vi "edit1.vi"() -> ()   [LabVIEW 2017]
uses:
  <vilib>/userdefined/High Color/IMAQdx.ctl
  <vilib>/myRIO/Instrument Drivers/Onboard IO/DIO/typedefs/DIO Reference.ctl
  <vilib>/myRIO/Common/Instrument Driver Framework/Utilities/typedefs/myRIO Generic Hardware Reference.ctl
  <vilib>/myRIO/Common/Instrument Driver Framework/Utilities/typedefs/Hardware Version Enum.ctl
  <vilib>/myRIO/Common/Instrument Driver Framework/Utilities/typedefs/myRIO v1.0 Reference.ctl
  <vilib>/myRIO/Common/Instrument Driver Framework/Utilities/typedefs/Generic FPGA Reference.ctl
  <vilib>/myRIO/Common/Instrument Driver Framework/myRIO v1.0/DIO/typedefs/DIO Channels List.ctl
  <vilib>/myRIO/Common/Instrument Driver Framework/myRIO v1.0/DIO/typedefs/DIO Channels Enum.ctl
  <vilib>/userdefined/High Color/nirio_resource_hc.ctl
  <vilib>/Platform/TimedLoop/XDataNode/timing_clust.ctl
  <vilib>/Platform/TimedLoop/XDataNode/nitl_modes.ctl
  <vilib>/Platform/TimedLoop/XDataNode/wakeup.ctl
  <vilib>/myRIO/Common/Instrument Driver Framework/Utilities/vis/Is FPGA Ref Available.vi
  <vilib>/myRIO/Common/Instrument Driver Framework/myRIO v1.0/DIO/vis/myRIO v1.1 Open DIO.vi
  <vilib>/myRIO/Instrument Drivers/Onboard IO/DIO/vis/Read.vi
  <vilib>/myRIO/Common/Instrument Driver Framework/Utilities/vis/Validate Channels.vi
  <vilib>/myRIO/Common/Instrument Driver Framework/myRIO v1.0/DIO/vis/myRIO v1.0 Reserve DIO.vi
  <vilib>/myRIO/Common/Instrument Driver Framework/myRIO v1.0/UART/vis/myRIO v1.0 Close UART.vi
  <vilib>/myRIO/Common/Instrument Driver Framework/myRIO v1.0/Resource Manager/vis/myRIO v1.0 Reserve Channel List.vi
  <vilib>/myRIO/Common/Instrument Driver Framework/myRIO v1.0/DIO/vis/myRIO v1.0 Build MUX Configuration DIO.vi
  <vilib>/myRIO/Common/Instrument Driver Framework/myRIO v1.0/Resource Manager/vis/myRIO v1.0 Reserve Channel.vi
  <vilib>/myRIO/Common/Instrument Driver Framework/myRIO v1.0/Resource Manager/vis/myRIO v1.0 Unreserve Channel.vi
  <vilib>/myRIO/Common/Instrument Driver Framework/myRIO v1.0/Resource Manager/vis/myRIO v1.0 Create Configuration List.vi
  <vilib>/myRIO/Common/Instrument Driver Framework/myRIO v1.0/Resource Manager/vis/myRIO v1.0 Build Mutex Name.vi
  Global 1.vi
  Outputs.vi
  Inputs.vi
  <vilib>/Utility/VariantDataType/GetNumericInfo.vi
  <vilib>/Utility/error.llb/Error Cluster From Error Code.vi
  <vilib>/myRIO/Common/Instrument Driver Framework/myRIO v1.0/myRIO v1.1 Open.vi
  <vilib>/myRIO/Common/Instrument Driver Framework/Utilities/vis/IO Manager.vi
  <vilib>/myRIO/Common/Instrument Driver Framework/Utilities/vis/Configuration Manager.vi
  <vilib>/myRIO/Common/Instrument Driver Framework/myRIO v1.0/Resource Manager/vis/myRIO v1.0 Configure IO.vi
  <vilib>/myRIO/Common/Instrument Driver Framework/myRIO v1.0/myRIO v1.0 Close.vi
  <vilib>/myRIO/Common/Instrument Driver Framework/myRIO v1.0/DIO/vis/myRIO v1.0 Read DIO.vi
  <vilib>/myRIO/Common/Instrument Driver Framework/Utilities/vis/FPGA Ref Manager.vi
  <vilib>/myRIO/Common/Instrument Driver Framework/myRIO v1.0/myRIO v1.0 Reset FPGA.vi
  <vilib>/myRIO/Common/Instrument Driver Framework/myRIO v1.0/IRQ/vis/myRIO v1.0 IRQ Info FGV.vi
  <vilib>/myRIO/Common/Instrument Driver Framework/myRIO v1.0/IRQ/vis/myRIO v1.0 Timer IRQ Info FGV.vi
  <vilib>/myRIO/Common/Instrument Driver Framework/myRIO v1.0/IRQ/vis/myRIO v1.0 ISR Agent.vi
  <vilib>/myRIO/Express VI/Onboard IO/DI/DI Express VI.xnode
  <vilib>/myRIO/Instrument Drivers/Onboard IO/DIO/vis/myRIO DIO Open.xnode
  <vilib>/platform/TimedLoop/XDataNode/XDataNode.xnode
  <vilib>/vision/driver/NI_Vision_Acquisition_Software.lvlib
  <vilib>/Platform/TimedLoop/XDataNode/XDNodeRunTimeDep.lvlib
  <vilib>/myRIO/Instrument Drivers/Utilities/Utilities.lvlib
  <vilib>/myRIO/Instrument Drivers/Onboard IO/DIO/DIO.lvlib
panel:
  out "error out":errorcluster
  in  "Stop":bool
  out "Step":i16
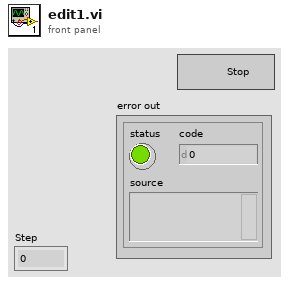
[diagram p1: front panel]
types:
  T1 = typedef "IMAQdx.ctl" = refnum<k21>
  T2 = typedef "DIO.lvlib/DIO Reference.ctl" = cluster{"myRIO Reference":T3, "DIO Channels List":T7}
  T3 = typedef "myRIO Generic Hardware Reference.ctl" = cluster{"myRIO Model":T4, "myRIO Hardware Reference":T5}
  T4 = typedef "Hardware Version Enum.ctl" = enum16{"Unknown", "myRIO-1900", "myRIO-1950", "roboRIO", "NI ELVIS RIO CM"}
  T5 = typedef "myRIO v1.0 Reference.ctl" = cluster{"Generic FPGA Reference":T6, "Allow multiple opens":bool}
  T6 = typedef "Generic FPGA Reference.ctl" = refnum<k20>
  T7 = typedef "DIO Channels List.ctl" = T8[]
  T8 = typedef "DIO Channels Enum.ctl" = enum16{"Not Connected", "C/DIO0", "C/DIO1", "C/DIO2", "C/DIO3", "C/DIO4", "C/DIO5", "C/DIO6", "C/DIO7", "A/DIO0", "A/DIO1", "A/DIO2", "A/DIO3", "A/DIO4", "A/DIO5", "A/DIO6", "A/DIO7", "A/DIO8", "A/DIO9", "A/DIO10", "A/DIO11", "A/DIO12", "A/DIO13", "A/DIO14", "A/DIO15", "B/DIO0", "B/DIO1", "B/DIO2", "B/DIO3", "B/DIO4", "B/DIO5", "B/DIO6", "B/DIO7", "B/DIO8", "B/DIO9", "B/DIO10", "B/DIO11", "B/DIO12", "B/DIO13", "B/DIO14", "B/DIO15", "LED0", "LED1", "LED2", "LED3", "Button0", "DIO/DIO0", "DIO/DIO1", "DIO/DIO2", "DIO/DIO3", "DIO/DIO4", "DIO/DIO5", "DIO/DIO6", "DIO/DIO7", "DIO/DIO8", "DIO/DIO9", "SPI/CS0", "SPI/CS1", "SPI/CS2", "SPI/CS3", "LED RADIO (Green)", "LED RADIO (Red)", "LED COMM (Green)", "LED COMM (Red)", "LED MODE (Green)", "LED MODE (Red)"}
  T9 = typedef "nirio_resource_hc.ctl" = tag
  T10 = typedef "XDNodeRunTimeDep.lvlib/timing_clust.ctl" = cluster{"Expected End [f-1]":u64, "Actual End [f-1]":u64, "Finished Late? [f-1]":bool, "Expected End [i-1]":u64, "Actual End [i-1]":u64, "Finished Late? [i-1]":bool, "Expected Start [i]":u64, "Actual Start [i]":u64, "Expected Start [f]":u64, "Actual Start [f]":u64, "Source Name":string, "Structure Name":string, "Period":i64, "Deadline":i64, "Offset":i64, "Start":i64, "Priority":i32, "Timeout":i32, "Mode":T11, "Wakeup Reason":T12, "Error":errorcluster, "Source Type":string, "Secondary Source Type":string, "Global End Time":u64, "Global Start Time":u64, "Frame Duration":u64, "Iteration Duration":u64, "Assigned CPU":i32, "I/O Scan Engine Mode":u32}
  T11 = typedef "XDNodeRunTimeDep.lvlib/nitl_modes.ctl" = enum32{"No Change", "Process missed periods, maintain original phase", "Discard missed periods, maintain original phase", "Process missed periods, ignore original phase", "Discard missed periods, ignore original phase"}
  T12 = typedef "XDNodeRunTimeDep.lvlib/wakeup.ctl" = enum32{"Normal", "Aborted", "Asynchronous wakeup", "Timing source error", "Timed loop error", "Timeout"}
  T13 = typedef "I2C.lvlib/I2C Reference.ctl" = cluster{"myRIO Reference":T3, "I2C Channels Enum":T14, "I2C Configuration":T15}
  T14 = typedef "I2C Channels Enum.ctl" = enum16{"Not Connected", "A/I2C", "B/I2C", "I2C/I2C"}
  T15 = typedef "I2C.lvlib/I2C Configuration.ctl" = cluster{"I2C Transfer Rate":T16}
  T16 = typedef "I2C.lvlib/I2C Transfer Rate.ctl" = enum16{"Standard mode (100 kbps)", "Fast mode (400 kbps)"}
  T17 = typedef "IMAQ Image.ctl" = refnum<image>
  T18 = typedef "IMAQ GM Match Report.ctl" = cluster{"Position":cluster{"x":sgl, "y":sgl}, "Angle":sgl, "Scale":sgl, "Score":sgl, "Bounding Box":cluster{"x":sgl, "y":sgl}[], "Contrast Reversed":bool, "Occlusion %":sgl, "Template Target Curve Score":sgl, "Target Template Curve Score":sgl, "Correlation Score":sgl}
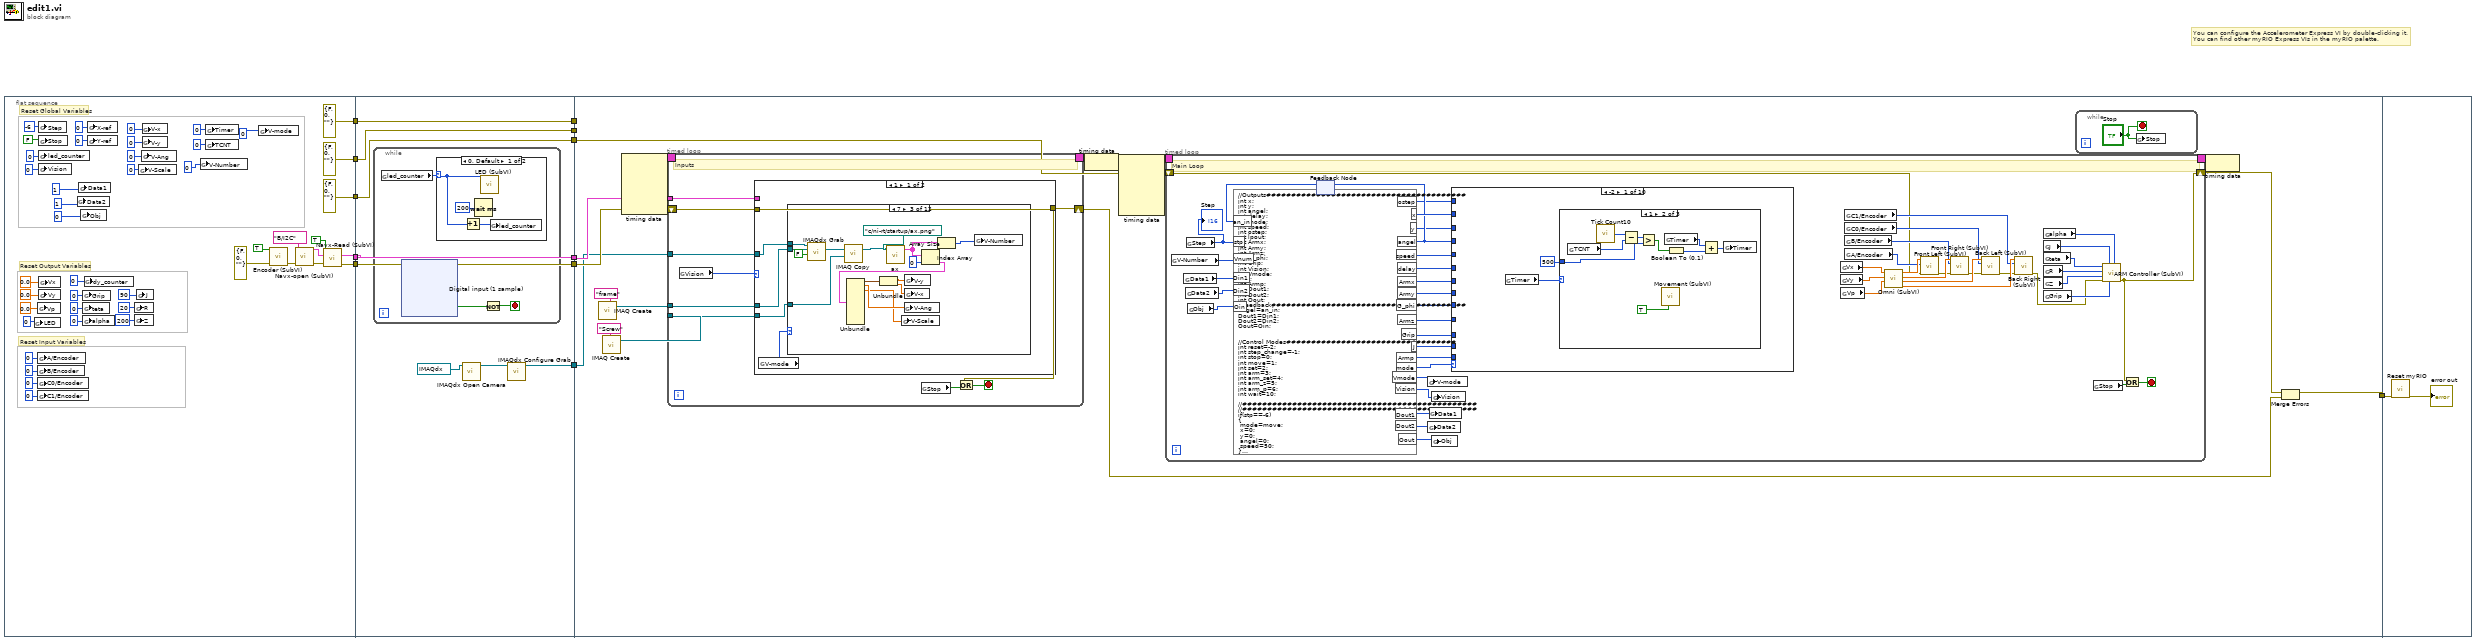
[diagram p0: block diagram]
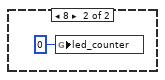
[diagram p2: hidden frame]
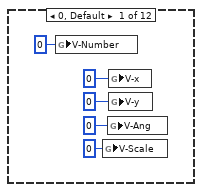
[diagram p3: hidden frame]
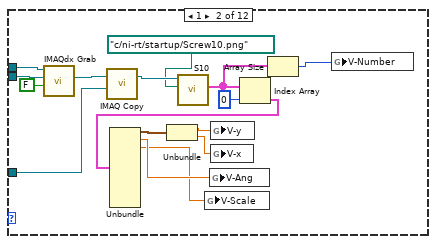
[diagram p4: hidden frame]
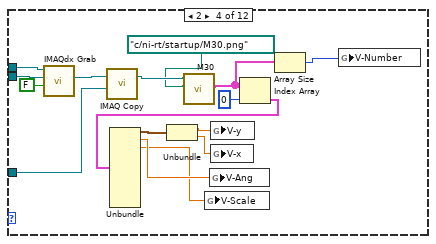
[diagram p5: hidden frame]
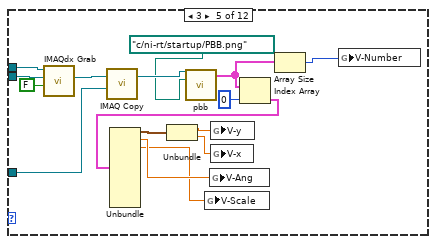
[diagram p6: hidden frame]
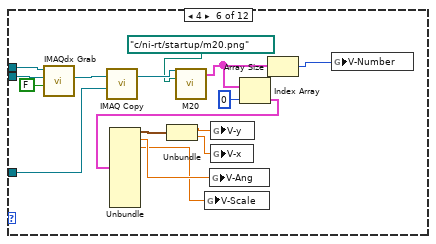
[diagram p7: hidden frame]
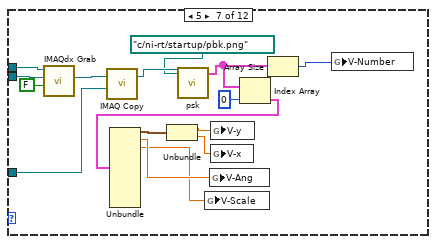
[diagram p8: hidden frame]
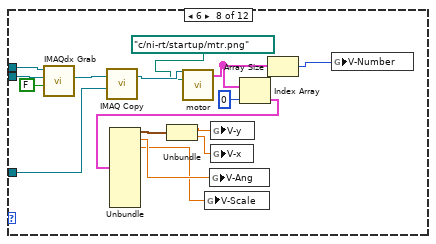
[diagram p9: hidden frame]
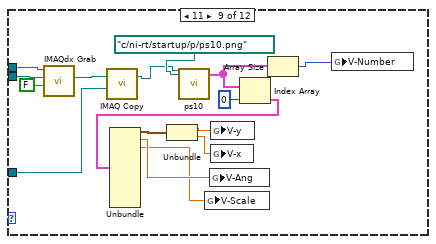
[diagram p10: hidden frame]
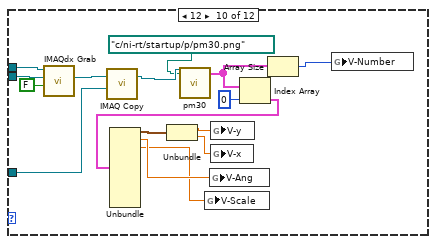
[diagram p11: hidden frame]
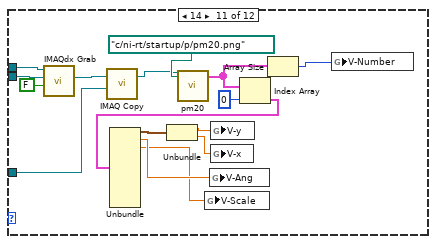
[diagram p12: hidden frame]
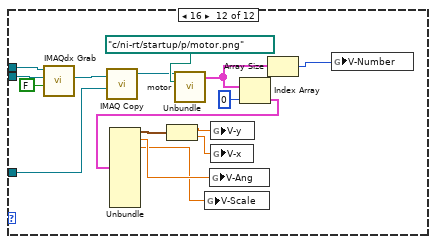
[diagram p13: hidden frame]
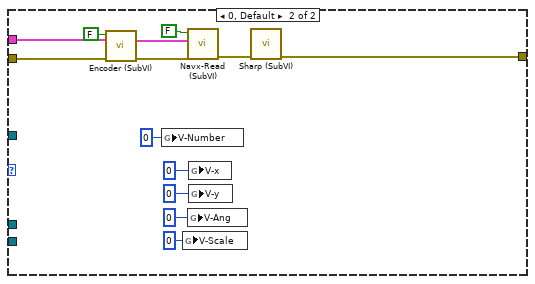
[diagram p14: hidden frame]
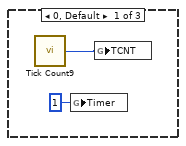
[diagram p15: hidden frame]
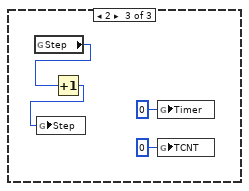
[diagram p16: hidden frame]
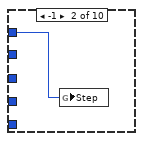
[diagram p17: hidden frame]
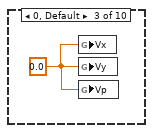
[diagram p18: hidden frame]
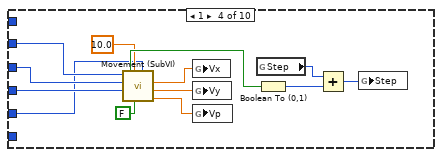
[diagram p19: hidden frame]
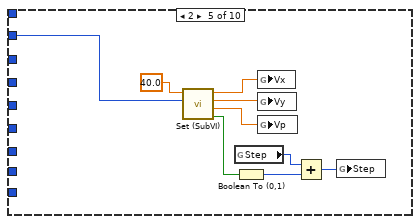
[diagram p20: hidden frame]
diagram:
  # "You can configure the Accelerometer Express VI by double-clicking it.\nYou can find other myRIO Express VIs in the myRIO palette."
  n1 = flat-sequence {
    tunnel: [w51] -> w12
    tunnel: [errorcluster {"status"=FALSE, "code"=0, "source"=""} ("error in (no error)")] -> w11
    tunnel: [errorcluster {"status"=FALSE, "code"=0, "source"=""} ("error in (no error)")] -> w10
    tunnel: [w49] -> w9
    tunnel: [errorcluster {"status"=FALSE, "code"=0, "source"=""} ("error in (no error)")] -> w8
    tunnel: w12 -> [w63]
    tunnel: [w63] -> w7
    tunnel: w11 -> [w62]
    tunnel: [w62] -> w6
    tunnel: w10 -> [w59]
    tunnel: w9 -> [w61]
    tunnel: [w61] -> w5
    tunnel: [w60] -> w4
    tunnel: w8 -> [w60]
    tunnel: [w59] -> w3
    tunnel: [w56] -> w2
    tunnel: w7 -> [w120]
    tunnel: w6 -> [_]
    tunnel: w5 -> [w115]
    tunnel: w4 -> [_]
    tunnel: [w114] -> w1
    tunnel: w3 -> [w111]
    tunnel: w2 -> [w110]
    tunnel: w1 -> [w545]
    frame #0 {
      # "Reset Global Variables"
      # "Reset Input Variables"
      # "Reset Output Variables"
      # "Initialize"
      n2 = global write "Outputs.vi" "LED"(i8 0 ("LED")) -> ()
      n3 = global write "Outputs.vi" "Vp"(0.0 ("Vp")) -> ()
      n4 = global write "Inputs.vi" "A/Encoder"(0 ("A/Encoder")) -> ()
      n5 = global write "Inputs.vi" "B/Encoder"(0 ("B/Encoder")) -> ()
      n6 = global write "Inputs.vi" "C0/Encoder"(0 ("C0/Encoder")) -> ()
      n7 = global write "Inputs.vi" "C1/Encoder"(0 ("C1/Encoder")) -> ()
      n8 = global write "Global 1.vi" "Step"(i16 -6 ("Step")) -> ()
      n9 = global write "Global 1.vi" "led_counter"(i8 0 ("Step")) -> ()
      n10 = global write "Global 1.vi" "Vision"(i8 0 ("Step")) -> ()
      n11 = global write "Outputs.vi" "Vy"(0.0 ("Vy")) -> ()
      n12 = global write "Global 1.vi" "Stop"(FALSE ("Stop")) -> ()
      n13 = global write "Outputs.vi" "Vx"(0.0 ("Vx")) -> ()
      n14 = global write "Global 1.vi" "Data2"(i16 1 ("Data2")) -> ()
      n15 = global write "Global 1.vi" "Data1"(i16 1 ("Data1")) -> ()
      n16 = global write "Global 1.vi" "Obj"(i16 0 ("Obj")) -> ()
      n17 = global write "Outputs.vi" "Grip"(i16 0 ("Grip")) -> ()
      n18 = global write "Outputs.vi" "teta"(i16 0 ("teta")) -> ()
      n19 = global write "Outputs.vi" "alpha"(i16 0 ("alpha")) -> ()
      n20 = global write "Outputs.vi" "dy_counter"(i8 0 ("LED")) -> ()
      n21 = global write "Global 1.vi" "X-ref"(i64 0 ("X-ref")) -> ()
      n22 = global write "Global 1.vi" "Y-ref"(i64 0 ("Y-ref")) -> ()
      n23 = global write "Outputs.vi" "R"(i16 20 ("R")) -> ()
      n24 = global write "Outputs.vi" "Z"(i16 200 ("Z")) -> ()
      n25 = global write "Outputs.vi" "J"(i16 90 ("J")) -> ()
      n26 = global write "Global 1.vi" "V-Scale"(i64 0 ("Y-ref")) -> ()
      n27 = global write "Global 1.vi" "V-Ang"(i64 0 ("X-ref")) -> ()
      n28 = global write "Global 1.vi" "V-x"(i64 0 ("X-ref")) -> ()
      n29 = global write "Global 1.vi" "V-y"(i64 0 ("Y-ref")) -> ()
      n30 = global write "Global 1.vi" "V-Number"(u8 0 ("V-Number")) -> ()
      n31 = global write "Global 1.vi" "Timer"(i16 0 ("Timer")) -> ()
      n32 = global write "Global 1.vi" "TCNT"(i16 0 ("Timer")) -> ()
      n33 = global write "Global 1.vi" "V-mode"(u8 0 ("V-Number")) -> ()
      n34 = call "Encoder (SubVI).vi"("error in (no error)"=errorcluster {"status"=FALSE, "code"=0, "source"=""}, "Reset?"=TRUE ("Reset Counter")) -> ("error out"=w33:errorcluster)  [unwired: 9 in]
      n35 = call "Navx-open (SubVI).vi"("error in (no error)"=w33, "Channel Name"=tag "B/I2C") -> ("error out"=w53:errorcluster, "I2C Ref Out"=w49:T13)  [unwired: 8 in]
      n36 = call "Navx-Read (SubVI).vi"("error in (no error)"=w53, "I2C Ref Out"=w49, "Reset"=TRUE) -> ("error out"=w51:errorcluster)  [unwired: 7 in, 1 out]
    }
    frame #1 {
      n37 = while {
        stop <- w65 stop-if-true
        n38 = global read "Global 1.vi" "led_counter"() -> (w66:i8)
        n39 = xnode "Digital input (1 sample)"() -> ("A/DIO15 (Pin 34)"=w64:bool)  [unwired: 1 in, 1 out]
        n40 = case shown="0, Default" w66 {
          selector: w66 -> [w102 _]
          frame 0, Default {
            n41 = Increment(x=w102) -> (x+1=w104:i8)
            n42 = Wait (ms)(milliseconds to wait=u32 200) -> ()  [unwired: 1 out]
            n43 = call "LED (SubVI).vi"("LED"=w102) -> ()  [unwired: 10 in, 1 out]
            n44 = global write "Global 1.vi" "led_counter"(w104) -> ()
          }
          frame 8 {
            n45 = global write "Global 1.vi" "led_counter"(i8 0 ("led_counter")) -> ()
          }
        }
        n46 = Not(x=w64) -> (.not. x?=w65:bool)
      }
      n47 = call <vilib>:"IMAQdx Open Camera.vi"("Session In"=T1 "cam0") -> ("Session Out"=w57:T1)  [unwired: 9 in, 1 out]
      n48 = call <vilib>:"IMAQdx Configure Grab.vi"("Session In"=w57) -> ("Session Out"=w56:T1)  [unwired: 9 in, 1 out]
    }
    frame #2 {
      n49 = call "IMAQ Create"("Image Name"="frame") -> ("New Image"=w107:T17)  [unwired: 4 in, 1 out]
      n50 = call "IMAQ Create"("Image Name"="Screw") -> ("New Image"=w106:T17)  [unwired: 4 in, 1 out]
      n51 = node-c288() -> (w117:T10)  [unwired: 5 in]
      n52 = timed-loop {
        shift-right: [w125] -> w113
        shift-left: w120 -> [w129]
        timing: w117 -> [_]
        timing-out: [_] -> w116
        tunnel: w115 -> [w127]
        tunnel: w110 -> [w123]
        tunnel: w107 -> [w122]
        tunnel: w106 -> [w121]
        stop <- w128 stop-if-true
        # "Inputs"
        n53 = global read "Global 1.vi" "Vision"() -> (w124:i16)
        n54 = case shown="1" w124 {
          tunnel: w129 -> [w131 w327]
          tunnel: w127 -> [_ w324]
          tunnel: [w131 w322] -> w125
          tunnel: w123 -> [w134 _]
          tunnel: w122 -> [w133 _]
          tunnel: w121 -> [w132 _]
          frame 1 {
            n55 = global read "Global 1.vi" "V-mode"() -> (w130:i16)
            n56 = case shown="7" w130 {
              tunnel: w133 -> [_ w153 w170 w186 w202 w218 w234 w250 w266 w282 w298 w314]
              tunnel: w132 -> [_ w152 w169 w185 w201 w217 w233 w249 w265 w281 w297 w313]
              tunnel: w134 -> [_ w143 w161 w177 w193 w209 w225 w241 w257 w273 w289 w305]
              frame 0, Default {
                n57 = global write "Global 1.vi" "V-Number"(u8 0 ("V-Number")) -> ()
                n58 = global write "Global 1.vi" "V-Scale"(i64 0 ("Y-ref")) -> ()
                n59 = global write "Global 1.vi" "V-Ang"(i64 0 ("X-ref")) -> ()
                n60 = global write "Global 1.vi" "V-x"(i64 0 ("X-ref")) -> ()
                n61 = global write "Global 1.vi" "V-y"(i64 0 ("Y-ref")) -> ()
              }
              frame 1 {
                n62 = call <vilib>:"IMAQdx Grab.vi"("Wait for Next Buffer? (Yes)"=FALSE, "Image In"=w153, "Session In"=w143) -> ("Image Out"=w155:T17)  [unwired: 5 in, 3 out]
                n63 = call "IMAQ Copy"("Image Dst"=w152, "Image Src"=w155) -> ("Image Dst Out"=w154:T17)  [unwired: 4 in, 1 out]
                n64 = call "S10.vi"("Template File Path (Geometric Matching 1)"=path "c:/ni-rt/startup/Screw10.png", "Image In"=w154) -> ("Matches (Geometric Matching 1)"=w141:T18[])  [unwired: 5 in, 2 out]
                n65 = Index Array(array=w141, index=0) -> (element=w149:T18)
                n66 = Unbundle(w149) -> ("Position"=w148:cluster{"x":sgl, "y":sgl}, "Angle"=w145:sgl, "Scale"=w144:sgl)  [unwired: 7 out]
                n67 = Unbundle(w148) -> ("x"=w147:sgl, "y"=w146:sgl)
                n68 = global write "Global 1.vi" "V-Scale"(w144) -> ()
                n69 = global write "Global 1.vi" "V-Ang"(w145) -> ()
                n70 = global write "Global 1.vi" "V-y"(w147) -> ()
                n71 = global write "Global 1.vi" "V-x"(w146) -> ()
                n72 = Array Size(array=w141) -> (size(s)=w140:i32)
                n73 = global write "Global 1.vi" "V-Number"(w140) -> ()
              }
              frame 7 {
                n74 = call <vilib>:"IMAQdx Grab.vi"("Wait for Next Buffer? (Yes)"=FALSE, "Image In"=w170, "Session In"=w161) -> ("Image Out"=w171:T17)  [unwired: 5 in, 3 out]
                n75 = call "IMAQ Copy"("Image Dst"=w169, "Image Src"=w171) -> ("Image Dst Out"=w156:T17)  [unwired: 4 in, 1 out]
                n76 = call "ax.vi"("Image In"=w156, "Template File Path (Geometric Matching 1)"=path "c:/ni-rt/startup/ax.png") -> ("Matches (Geometric Matching 1)"=w158:T18[])  [unwired: 23 in, 2 out]
                n77 = Index Array(array=w158, index=0) -> (element=w167:T18)
                n78 = Unbundle(w167) -> ("Position"=w166:cluster{"x":sgl, "y":sgl}, "Angle"=w163:sgl, "Scale"=w162:sgl)  [unwired: 7 out]
                n79 = Unbundle(w166) -> ("x"=w165:sgl, "y"=w164:sgl)
                n80 = global write "Global 1.vi" "V-Scale"(w162) -> ()
                n81 = global write "Global 1.vi" "V-Ang"(w163) -> ()
                n82 = global write "Global 1.vi" "V-y"(w165) -> ()
                n83 = global write "Global 1.vi" "V-x"(w164) -> ()
                n84 = Array Size(array=w158) -> (size(s)=w159:i32)
                n85 = global write "Global 1.vi" "V-Number"(w159) -> ()
              }
              frame 2 {
                n86 = call <vilib>:"IMAQdx Grab.vi"("Wait for Next Buffer? (Yes)"=FALSE, "Image In"=w186, "Session In"=w177) -> ("Image Out"=w187:T17)  [unwired: 5 in, 3 out]
                n87 = call "IMAQ Copy"("Image Dst"=w185, "Image Src"=w187) -> ("Image Dst Out"=w176:T17)  [unwired: 4 in, 1 out]
                n88 = call "M30.vi"("Template File Path (Geometric Matching 1)"=path "c:/ni-rt/startup/M30.png", "Image In"=w176) -> ("Matches (Geometric Matching 1)"=w172:T18[])  [unwired: 3 in, 2 out]
                n89 = Index Array(array=w172, index=0) -> (element=w183:T18)
                n90 = Unbundle(w183) -> ("Position"=w182:cluster{"x":sgl, "y":sgl}, "Angle"=w179:sgl, "Scale"=w178:sgl)  [unwired: 7 out]
                n91 = Unbundle(w182) -> ("x"=w181:sgl, "y"=w180:sgl)
                n92 = global write "Global 1.vi" "V-Scale"(w178) -> ()
                n93 = global write "Global 1.vi" "V-Ang"(w179) -> ()
                n94 = global write "Global 1.vi" "V-y"(w181) -> ()
                n95 = global write "Global 1.vi" "V-x"(w180) -> ()
                n96 = Array Size(array=w172) -> (size(s)=w173:i32)
                n97 = global write "Global 1.vi" "V-Number"(w173) -> ()
              }
              frame 3 {
                n98 = call <vilib>:"IMAQdx Grab.vi"("Wait for Next Buffer? (Yes)"=FALSE, "Image In"=w202, "Session In"=w193) -> ("Image Out"=w203:T17)  [unwired: 5 in, 3 out]
                n99 = call "IMAQ Copy"("Image Dst"=w201, "Image Src"=w203) -> ("Image Dst Out"=w190:T17)  [unwired: 4 in, 1 out]
                n100 = call "pbb.vi"("Image In"=w190, "Template File Path (Geometric Matching 1)"=path "c:/ni-rt/startup/PBB.png") -> ("Calibrated Matches (Geometric Matching 1)"=w188:T18[])  [unwired: 23 in, 2 out]
                n101 = Index Array(array=w188, index=0) -> (element=w199:T18)
                n102 = Unbundle(w199) -> ("Position"=w198:cluster{"x":sgl, "y":sgl}, "Angle"=w195:sgl, "Scale"=w194:sgl)  [unwired: 7 out]
                n103 = Unbundle(w198) -> ("x"=w197:sgl, "y"=w196:sgl)
                n104 = global write "Global 1.vi" "V-Scale"(w194) -> ()
                n105 = global write "Global 1.vi" "V-Ang"(w195) -> ()
                n106 = global write "Global 1.vi" "V-y"(w197) -> ()
                n107 = global write "Global 1.vi" "V-x"(w196) -> ()
                n108 = Array Size(array=w188) -> (size(s)=w191:i32)
                n109 = global write "Global 1.vi" "V-Number"(w191) -> ()
              }
              frame 4 {
                n110 = call <vilib>:"IMAQdx Grab.vi"("Wait for Next Buffer? (Yes)"=FALSE, "Image In"=w218, "Session In"=w209) -> ("Image Out"=w219:T17)  [unwired: 5 in, 3 out]
                n111 = call "IMAQ Copy"("Image Dst"=w217, "Image Src"=w219) -> ("Image Dst Out"=w205:T17)  [unwired: 4 in, 1 out]
                n112 = call "M20.vi"("Image In"=w205, "Template File Path (Geometric Matching 1)"=path "c:/ni-rt/startup/m20.png") -> ("Calibrated Matches (Geometric Matching 1)"=w206:T18[])  [unwired: 23 in, 2 out]
                n113 = Index Array(array=w206, index=0) -> (element=w215:T18)
                n114 = Unbundle(w215) -> ("Position"=w214:cluster{"x":sgl, "y":sgl}, "Angle"=w211:sgl, "Scale"=w210:sgl)  [unwired: 7 out]
                n115 = Unbundle(w214) -> ("x"=w213:sgl, "y"=w212:sgl)
                n116 = global write "Global 1.vi" "V-Scale"(w210) -> ()
                n117 = global write "Global 1.vi" "V-Ang"(w211) -> ()
                n118 = global write "Global 1.vi" "V-y"(w213) -> ()
                n119 = global write "Global 1.vi" "V-x"(w212) -> ()
                n120 = Array Size(array=w206) -> (size(s)=w207:i32)
                n121 = global write "Global 1.vi" "V-Number"(w207) -> ()
              }
              frame 5 {
                n122 = call <vilib>:"IMAQdx Grab.vi"("Wait for Next Buffer? (Yes)"=FALSE, "Image In"=w234, "Session In"=w225) -> ("Image Out"=w235:T17)  [unwired: 5 in, 3 out]
                n123 = call "IMAQ Copy"("Image Dst"=w233, "Image Src"=w235) -> ("Image Dst Out"=w221:T17)  [unwired: 4 in, 1 out]
                n124 = call "psk.vi"("Image In"=w221, "Template File Path (Geometric Matching 1)"=path "c:/ni-rt/startup/pbk.png") -> ("Matches (Geometric Matching 1)"=w222:T18[])  [unwired: 23 in, 2 out]
                n125 = Index Array(array=w222, index=0) -> (element=w231:T18)
                n126 = Unbundle(w231) -> ("Position"=w230:cluster{"x":sgl, "y":sgl}, "Angle"=w227:sgl, "Scale"=w226:sgl)  [unwired: 7 out]
                n127 = Unbundle(w230) -> ("x"=w229:sgl, "y"=w228:sgl)
                n128 = global write "Global 1.vi" "V-Scale"(w226) -> ()
                n129 = global write "Global 1.vi" "V-Ang"(w227) -> ()
                n130 = global write "Global 1.vi" "V-y"(w229) -> ()
                n131 = global write "Global 1.vi" "V-x"(w228) -> ()
                n132 = Array Size(array=w222) -> (size(s)=w223:i32)
                n133 = global write "Global 1.vi" "V-Number"(w223) -> ()
              }
              frame 6 {
                n134 = call <vilib>:"IMAQdx Grab.vi"("Wait for Next Buffer? (Yes)"=FALSE, "Image In"=w250, "Session In"=w241) -> ("Image Out"=w251:T17)  [unwired: 5 in, 3 out]
                n135 = call "IMAQ Copy"("Image Dst"=w249, "Image Src"=w251) -> ("Image Dst Out"=w237:T17)  [unwired: 4 in, 1 out]
                n136 = call "motor.vi"("Image In"=w237, "Template File Path (Geometric Matching 1)"=path "c:/ni-rt/startup/mtr.png") -> ("Calibrated Matches (Geometric Matching 1)"=w238:T18[])  [unwired: 23 in, 2 out]
                n137 = Index Array(array=w238, index=0) -> (element=w247:T18)
                n138 = Unbundle(w247) -> ("Position"=w246:cluster{"x":sgl, "y":sgl}, "Angle"=w243:sgl, "Scale"=w242:sgl)  [unwired: 7 out]
                n139 = Unbundle(w246) -> ("x"=w245:sgl, "y"=w244:sgl)
                n140 = global write "Global 1.vi" "V-Scale"(w242) -> ()
                n141 = global write "Global 1.vi" "V-Ang"(w243) -> ()
                n142 = global write "Global 1.vi" "V-y"(w245) -> ()
                n143 = global write "Global 1.vi" "V-x"(w244) -> ()
                n144 = Array Size(array=w238) -> (size(s)=w239:i32)
                n145 = global write "Global 1.vi" "V-Number"(w239) -> ()
              }
              frame 11 {
                n146 = call <vilib>:"IMAQdx Grab.vi"("Wait for Next Buffer? (Yes)"=FALSE, "Image In"=w266, "Session In"=w257) -> ("Image Out"=w267:T17)  [unwired: 5 in, 3 out]
                n147 = call "IMAQ Copy"("Image Dst"=w265, "Image Src"=w267) -> ("Image Dst Out"=w252:T17)  [unwired: 4 in, 1 out]
                n148 = call "ps10.vi"("Image In"=w252, "Template File Path (Geometric Matching 1)"=path "c:/ni-rt/startup/p/ps10.png") -> ("Matches (Geometric Matching 1)"=w254:T18[])  [unwired: 23 in, 2 out]
                n149 = Index Array(array=w254, index=0) -> (element=w263:T18)
                n150 = Unbundle(w263) -> ("Position"=w262:cluster{"x":sgl, "y":sgl}, "Angle"=w259:sgl, "Scale"=w258:sgl)  [unwired: 7 out]
                n151 = Unbundle(w262) -> ("x"=w261:sgl, "y"=w260:sgl)
                n152 = global write "Global 1.vi" "V-Scale"(w258) -> ()
                n153 = global write "Global 1.vi" "V-Ang"(w259) -> ()
                n154 = global write "Global 1.vi" "V-y"(w261) -> ()
                n155 = global write "Global 1.vi" "V-x"(w260) -> ()
                n156 = Array Size(array=w254) -> (size(s)=w255:i32)
                n157 = global write "Global 1.vi" "V-Number"(w255) -> ()
              }
              frame 12 {
                n158 = call <vilib>:"IMAQdx Grab.vi"("Wait for Next Buffer? (Yes)"=FALSE, "Image In"=w282, "Session In"=w273) -> ("Image Out"=w283:T17)  [unwired: 5 in, 3 out]
                n159 = call "IMAQ Copy"("Image Dst"=w281, "Image Src"=w283) -> ("Image Dst Out"=w269:T17)  [unwired: 4 in, 1 out]
                n160 = call "pm30.vi"("Image In"=w269, "Template File Path (Geometric Matching 1)"=path "c:/ni-rt/startup/p/pm30.png") -> ("Matches (Geometric Matching 1)"=w270:T18[])  [unwired: 23 in, 2 out]
                n161 = Index Array(array=w270, index=0) -> (element=w279:T18)
                n162 = Unbundle(w279) -> ("Position"=w278:cluster{"x":sgl, "y":sgl}, "Angle"=w275:sgl, "Scale"=w274:sgl)  [unwired: 7 out]
                n163 = Unbundle(w278) -> ("x"=w277:sgl, "y"=w276:sgl)
                n164 = global write "Global 1.vi" "V-Scale"(w274) -> ()
                n165 = global write "Global 1.vi" "V-Ang"(w275) -> ()
                n166 = global write "Global 1.vi" "V-y"(w277) -> ()
                n167 = global write "Global 1.vi" "V-x"(w276) -> ()
                n168 = Array Size(array=w270) -> (size(s)=w271:i32)
                n169 = global write "Global 1.vi" "V-Number"(w271) -> ()
              }
              frame 14 {
                n170 = call <vilib>:"IMAQdx Grab.vi"("Wait for Next Buffer? (Yes)"=FALSE, "Image In"=w298, "Session In"=w289) -> ("Image Out"=w299:T17)  [unwired: 5 in, 3 out]
                n171 = call "IMAQ Copy"("Image Dst"=w297, "Image Src"=w299) -> ("Image Dst Out"=w285:T17)  [unwired: 4 in, 1 out]
                n172 = call "pm20.vi"("Image In"=w285, "Template File Path (Geometric Matching 1)"=path "c:/ni-rt/startup/p/pm20.png") -> ("Matches (Geometric Matching 1)"=w284:T18[])  [unwired: 23 in, 2 out]
                n173 = Index Array(array=w284, index=0) -> (element=w295:T18)
                n174 = Unbundle(w295) -> ("Position"=w294:cluster{"x":sgl, "y":sgl}, "Angle"=w291:sgl, "Scale"=w290:sgl)  [unwired: 7 out]
                n175 = Unbundle(w294) -> ("x"=w293:sgl, "y"=w292:sgl)
                n176 = global write "Global 1.vi" "V-Scale"(w290) -> ()
                n177 = global write "Global 1.vi" "V-Ang"(w291) -> ()
                n178 = global write "Global 1.vi" "V-y"(w293) -> ()
                n179 = global write "Global 1.vi" "V-x"(w292) -> ()
                n180 = Array Size(array=w284) -> (size(s)=w287:i32)
                n181 = global write "Global 1.vi" "V-Number"(w287) -> ()
              }
              frame 16 {
                n182 = call <vilib>:"IMAQdx Grab.vi"("Wait for Next Buffer? (Yes)"=FALSE, "Image In"=w314, "Session In"=w305) -> ("Image Out"=w315:T17)  [unwired: 5 in, 3 out]
                n183 = call "IMAQ Copy"("Image Dst"=w313, "Image Src"=w315) -> ("Image Dst Out"=w300:T17)  [unwired: 4 in, 1 out]
                n184 = call "motor.vi"("Image In"=w300, "Template File Path (Geometric Matching 1)"=path "c:/ni-rt/startup/p/motor.png") -> ("Calibrated Matches (Geometric Matching 1)"=w302:T18[])  [unwired: 23 in, 2 out]
                n185 = Index Array(array=w302, index=0) -> (element=w311:T18)
                n186 = Unbundle(w311) -> ("Position"=w310:cluster{"x":sgl, "y":sgl}, "Angle"=w307:sgl, "Scale"=w306:sgl)  [unwired: 7 out]
                n187 = Unbundle(w310) -> ("x"=w309:sgl, "y"=w308:sgl)
                n188 = global write "Global 1.vi" "V-Scale"(w306) -> ()
                n189 = global write "Global 1.vi" "V-Ang"(w307) -> ()
                n190 = global write "Global 1.vi" "V-y"(w309) -> ()
                n191 = global write "Global 1.vi" "V-x"(w308) -> ()
                n192 = Array Size(array=w302) -> (size(s)=w303:i32)
                n193 = global write "Global 1.vi" "V-Number"(w303) -> ()
              }
            }
          }
          frame 0, Default {
            n194 = call "Encoder (SubVI).vi"("error in (no error)"=w327, "Reset?"=FALSE ("Boolean")) -> ("error out"=w325:errorcluster)  [unwired: 9 in]
            n195 = global write "Global 1.vi" "V-Number"(u8 0 ("V-Number")) -> ()
            n196 = global write "Global 1.vi" "V-Scale"(i64 0 ("Y-ref")) -> ()
            n197 = call "Navx-Read (SubVI).vi"("error in (no error)"=w325, "I2C Ref Out"=w324, "Reset"=FALSE) -> ("error out"=w323:errorcluster)  [unwired: 7 in, 1 out]
            n198 = global write "Global 1.vi" "V-Ang"(i64 0 ("X-ref")) -> ()
            n199 = global write "Global 1.vi" "V-x"(i64 0 ("X-ref")) -> ()
            n200 = global write "Global 1.vi" "V-y"(i64 0 ("Y-ref")) -> ()
            n201 = call "Sharp (SubVI).vi"("error in (no error)"=w323) -> ("error out"=w322:errorcluster)  [unwired: 10 in]
          }
        }
        n202 = global read "Global 1.vi" "Stop"() -> (w126:bool)
        n203 = Or(x=w125, y=w126) -> (x .or. y?=w128:bool)
      }
      n204 = node-c288(w116) -> ()
      n205 = node-c288() -> (w119:T10)  [unwired: 5 in]
      n206 = timed-loop {
        shift-right: [w341] -> w112
        shift-left: w111 -> [w343]
        timing: w119 -> [_]
        timing-out: [_] -> w118
        stop <- w381 stop-if-true
        # "Main Loop"
        n207 = global read "Global 1.vi" "V-Number"() -> (w340:u8)
        n208 = global read "Global 1.vi" "Data1"() -> (w337:i16)
        n209 = global read "Global 1.vi" "Data2"() -> (w336:i16)
        n210 = global read "Global 1.vi" "Step"() -> (w374:i16)
        "Step" <- w374
        n211 = global read "Global 1.vi" "Obj"() -> (w333:i16)
        n212 = feedback #1() -> (w378:i32)  [unwired: 1 in]
        n213 = formula code="//Outputs########################################\nint x;\nint y;\nint angel;\nint delay;\nint mode;\nint speed;\nint ostep;\nint lpout;\nint Armx;\nint Army;\nint Armz;\nint G_phi;\nint Grip;\nint Vision;\nint Vmode;\nint J;\nint Armp;\nint Dout1;\nint Dout2;\nint Oout;\n//Feedback#######################################\nangel=an_in;\nDout1=Din1;\nDout2=Din2;\nOout=Oin;\n\n\n//Control Modes##################################\nint reset=-2;\nint step_change=-1; \nint stop=0;\nint move=1;\nint set=2;\nint arm=3;\nint arm_set=4;\nint arm_z=5;\nint arm_p=6;\nint wait=10;\n\n//###############################################\n//###############################################\nif(stp==-6)\n{\n\tmode=move;\n\tx=0;\n\ty=0;\n\tangel=0;\n\tspeed=50;\n}\nif(stp==-5)\n{\n\tmode=move;\n\tx=450;\n\ty=0;\n\tangel=0;\n\tspeed=100;\n}\nif(stp==-4)\n{\n\tmode=move;\n\tx=0;\n\ty=-1500;\n\tangel=0;\n\tspeed=100;\n}\nif(stp==-3)\n{\n\tmode=move;\n\tx=1000;\n\ty=0;\n\tangel=0;\n\tspeed=100;\n}\nif(stp==-2)\n{\n\tmode=move;\n\tx=0;\n\ty=0;\n\tangel=-90;\n\tspeed=100;\n}\nif(stp==-1)\n{\n\tmode=set;\n\tx=1;\t\n}\nif(stp==0)\n{\n\tmode=reset;\n}\nif(stp==1)\n{\n\tmode=arm;\n\tArmx=75;\n\tArmy=0;\n\tArmz=280;\n\tJ=90;\n\tdelay=4000;\t\n}\n\n//Obj Search--------------------------\nif(stp==2)\n{\n\tmode=set;\n\tx=3;\n\tspeed=50;\n}\nif(stp==3)\n{\n\tmode=reset;\n}\n\n\nif(stp==4)\n{\n\tVision=1;\n\tVmode=7;\n\tif(Vnum==0)\n\t{\n\t\tmode=wait;\n\t\tdelay=1500;\n\t}\n\telse\n\t{\n\t\tDout1=1;\n\t\tDout2=Din2+1;\n\t\tmode=step_change;\n\t\tostep=500;\n\t}\n}\nif(stp==5)\n{\n\tVision=0;\n\tmode=reset;\n}\n\nif(stp==6)\n{\n\tmode=move;\n\tx=0;\n\ty=-250;\n\tangel=0;\n\tspeed=50;\n}\nif(stp==7)\n{\n\tmode=reset;\n}\nif(stp==8)\n{\n\tVision=1;\n\tVmode=7;\n\tif(Vnum==0)\n\t{\n\t\tmode=wait;\n\t\tdelay=1500;\n\t}\n\telse\n\t{\n\t\tDout1=2;\n\t\tDout2=Din2+1;\n\t\tmode=step_change;\n\t\tostep=500;\n\t}\n}\nif(stp==9)\n{\n\tVision=0;\n\tmode=reset;\n}\n\nif(stp==10)\n{\n\tmode=move;\n\tx=0;\n\ty=-250;\n\tangel=0;\n\tspeed=50;\n}\nif(stp==11)\n{\n\tmode=reset;\n}\nif(stp==12)\n{\n\tVision=1;\n\tVmode=7;\n\tif(Vnum==0)\n\t{\n\t\tmode=wait;\n\t\tdelay=1500;\n\t}\n\telse\n\t{\n\t\tDout1=3;\n\t\tDout2=Din2+1;\n\t\tmode=step_change;\n\t\tostep=500;\n\t}\n}\n\n\nif(stp==13)\n{\n\tVision=0;\n\tmode=reset;\n}\n\nif(stp==14)\n{\n\tmode=move;\n\tx=0;\n\ty=500;\n\tangel=0;\n\tspeed=100;\n}\n\nif(stp==15)\n{\n\tDout2=Din2+1;\n\tmode=step_change;\n\tostep=2;\n}\n\n//---------------------------\n\n\nif(stp==500)\n{\n\tmode=arm_set;\n\tArmx=75;\n\tArmy=0;\n\tdelay=2000;\n}\n\nif(stp==501)\n{\n\tmode=arm_z;\n\tArmz=100;\n\tGrip=0;\n\tdelay=3000;\n}\nif(stp==502)\n{\n\tmode=arm_z;\n\tArmz=100;\n\tGrip=1;\n\tdelay=1000;\n}\nif(stp==503)\n{\n\tmode=arm_z;\n\tArmz=200;\n\tGrip=1;\n\tdelay=1000;\n}\nif(stp==504)\n{\n\tmode=arm;\n\tArmx=20;\n\tArmy=0;\n\tArmz=200;\n\tGrip=1;\n\tJ=90;\n\tdelay=1000;\n}\nif(stp==505)\n{\n\tmode=reset;\n}\nif(stp==506) /////////deliver\n{\n\t\tmode=step_change;\n\t\tostep=507;\n}\n\n\nif(stp==507)\n{\n\tmode=arm_p;\n\tArmp=180;\n\tdelay=4000;\n}\n\nif(stp==508)\n{\n\tmode=arm_z;\n\tArmz=115;\n\tGrip=1;\n\tdelay=1500;\n}\nif(stp==509)\n{\n\tmode=arm_z;\n\tArmz=95;\n\tGrip=0;\n\tdelay=1000;\n}\nif(stp==510)\n{\n\tmode=reset;\n}\nif(stp==511) /////////deliver\n{\n\tmode=move;\n\tx=0;\n\ty=-1000;\n\tangel=0;\n\tspeed=100;\n}\nif(stp==512) \n{\n\tmode=move;\n\tx=500;\n\ty=0;\n\tangel=0;\n\tspeed=100;\n}\nif(stp==513)\n{\n\tmode=arm_z;\n\tArmz=95;\n\tGrip=1;\n\tdelay=1000;\n}\nif(stp==514)\n{\n\tmode=arm_z;\n\tArmz=115;\n\tGrip=1;\n\tdelay=1500;\n}\nif(stp==515)\n{\n\tmode=arm;\n\tArmx=-70;\n\tArmy=-400;\n\tArmz=120;\n\tGrip=1;\n\tJ=90;\n\tdelay=5000;\n}\nif(stp==516) \n{\n\tmode=move;\n\tx=0;\n\ty=-250;\n\tangel=0;\n\tspeed=100;\n}\n\nif(stp==517)\n{\n\tmode=arm_z;\n\tArmz=120;\n\tGrip=0;\n\tdelay=1500;\n}\nif(stp==518)\n{\n\tmode=arm_z;\n\tArmz=140;\n\tGrip=0;\n\tdelay=1000;\n}\nif(stp==519)\n{\n\tmode=arm;\n\tArmx=20;\n\tArmy=0;\n\tArmz=140;\n\tGrip=0;\n\tJ=90;\n\tdelay=2000;\n}\nif(stp==520) \n{\n\tmode=reset;\n}\n\nif(stp==521) \n{\n\tmode=move;\n\tx=0;\n\ty=-1000;\n\tangel=0;\n\tspeed=100;\n}\nif(stp==522) \n{\n\tmode=move;\n\tx=0;\n\ty=0;\n\tangel=90;\n\tspeed=100;\n}\nif(stp==523) \n{\n\tmode=move;\n\tx=1200;\n\ty=0;\n\tangel=0;\n\tspeed=100;\n}\nif(stp==524) \n{\n\tmode=move;\n\tx=0;\n\ty=-1500;\n\tangel=0;\n\tspeed=100;\n}\nif(stp==525)\n{\n\tmode=set;\n\tx=4;\n}\nif(stp==526)\n{\n\tmode=reset;\n}\nif(stp==527)\n{\n\tmode=move;\n\tx=2550;\n\ty=0;\n\tangel=0;\n\tspeed=100;\n}\nif(stp==528)\n{\n\tmode=arm;\n\tArmx=75;\n\tArmy=0;\n\tArmz=280;\n\tJ=90;\n\tdelay=4000;\t\n}\n\n//Obj Search--------------------------\nif(stp==529)\n{\n\tmode=step_change;\n\tostep=530;\n}\nif(stp==530)\n{\n\tmode=reset;\n}\n\n\nif(stp==531)\n{\n\tVision=1;\n\tVmode=7;\n\tif(Vnum!=0)\n\t{\n\t\tDout1=1;\n\t\tDout2=Din2+1;\n\t\tmode=step_change;\n\t\tostep=500;\n\t}\n}\n\n//---------------------------\n\n\nif(stp==532)\n{\n\tmode=arm_set;\n\tArmx=75;\n\tArmy=0;\n\tdelay=2000;\n}\n\nif(stp==533)\n{\n\tmode=arm_z;\n\tArmz=155;\n\tGrip=0;\n\tdelay=7000; ////00000000000000000000000000000000000000000000000000000000000000000000000/\n}\nif(stp==534)\n{\n\tmode=arm_z;\n\tArmz=100;\n\tGrip=2;\n\tdelay=1000;\n}\nif(stp==535)\n{\n\tmode=arm_z;\n\tArmz=100;\n\tGrip=0;\n\tdelay=500;\n}\nif(stp==536)\n{\n\tmode=arm_z;\n\tArmz=100;\n\tGrip=1;\n\tdelay=500;\n}\nif(stp==537)\n{\n\tmode=arm_z;\n\tArmz=200;\n\tGrip=1;\n\tdelay=1000;\n}\nif(stp==538)\n{\n\tmode=arm;\n\tArmx=20;\n\tArmy=0;\n\tArmz=200;\n\tGrip=1;\n\tJ=90;\n\tdelay=1000;\n}\n\nif(stp==539)\n{\n\tmode=arm_p;\n\tArmp=180;\n\tdelay=4000;\n}\nif(stp==540)\n{\n\tmode=arm_z;\n\tArmz=200;\n\tGrip=0;\n\tdelay=1000;\n}\n\nif(stp==541)\n{\n\tmode=arm;\n\tArmx=75;\n\tArmy=0;\n\tArmz=280;\n\tJ=90;\n\tdelay=4000;\t\n}\nif(stp==542)\n{\n\tmode=reset;\n}\n\n\nif(stp==543)\n{\n\tmode=stop;\n}"("stp"=w374, "an_in"=w378, "Vnum"=w340, "Din1"=w337, "Din2"=w336, "Oin"=w333) -> ("x"=w380:i32, "y"=w375:i32, "mode"=w364:i32, "angel"=w377:i32, "delay"=w379:i32, "speed"=w376:i32, "ostep"=w372:i32, "Armx"=w370:i32, "Army"=w369:i32, "Armz"=w368:i32, "G_phi"=w371:i32, "Grip"=w367:i32, "Vision"=w366:i32, "Vmode"=w365:i32, "J"=w339:i32, "Armp"=w338:i32, "Dout1"=w335:i32, "Dout2"=w334:i32, "Oout"=w332:i32)
        n214 = feedback-in #1(w377) -> ()
        n215 = global write "Global 1.vi" "V-mode"(w365) -> ()
        n216 = global write "Global 1.vi" "Data2"(w334) -> ()
        n217 = global write "Global 1.vi" "Data1"(w335) -> ()
        n218 = global write "Global 1.vi" "Vision"(w366) -> ()
        n219 = global write "Global 1.vi" "Obj"(w332) -> ()
        n220 = case shown="-2" w364 {
          tunnel: w380 -> [_ _ _ w407 w422 _ _ _ _ _]
          tunnel: w375 -> [_ _ _ w406 _ _ _ _ _ _]
          tunnel: w377 -> [_ _ _ w405 _ _ _ _ _ _]
          tunnel: w379 -> [_ _ _ _ _ w424 w460 w488 w507 w525]
          tunnel: w376 -> [_ _ _ w404 _ _ _ _ _ _]
          tunnel: w372 -> [_ w399 _ _ _ _ _ _ _ _]
          tunnel: w371 -> [_ _ _ _ _ w428 _ _ _ _]
          tunnel: w370 -> [_ _ _ _ _ w426 w455 _ _ _]
          tunnel: w369 -> [_ _ _ _ _ w427 w454 _ _ _]
          tunnel: w368 -> [_ _ _ _ _ w429 _ w487 _ _]
          tunnel: w367 -> [_ _ _ _ _ w425 _ w486 _ _]
          tunnel: w339 -> [_ _ _ _ _ w423 _ _ _ _]
          tunnel: w338 -> [_ _ _ _ _ _ _ _ w506 _]
          frame -2 {
            n221 = global read "Global 1.vi" "Timer"() -> (w382:i16)
            n222 = case shown="1" w382 {
              tunnel: 500 -> [_ w387 _]
              frame 0, Default {
                n223 = call "Tick Count9"() -> ("Tick Count(mSec)"=w385:u32)
                n224 = global write "Global 1.vi" "Timer"(i16 1 ("Timer")) -> ()
                n225 = global write "Global 1.vi" "TCNT"(w385) -> ()
              }
              frame 1 {
                n226 = global read "Global 1.vi" "TCNT"() -> (w392:u64)
                n227 = call "Tick Count10"() -> ("Tick Count(mSec)"=w394:u32)
                n228 = Subtract(x=w394, y=w392) -> (x-y=w393:u64)
                n229 = Greater?(x=w393, y=w387) -> (0:w388:bool)
                n230 = call "Movement (SubVI).vi"("Reset"=TRUE) -> ()  [unwired: 6 in, 4 out]
                n231 = global read "Global 1.vi" "Timer"() -> (w389:i16)
                n232 = Boolean To (0,1)(Boolean=w388) -> (0, 1=w391:i16)
                n233 = Add(x=w389, y=w391) -> (x+y=w390:i16)
                n234 = global write "Global 1.vi" "Timer"(w390) -> ()
              }
              frame 2 {
                n235 = global read "Global 1.vi" "Step"() -> (w397:i16)
                n236 = Increment(x=w397) -> (x+1=w398:i16)
                n237 = global write "Global 1.vi" "Step"(w398) -> ()
                n238 = global write "Global 1.vi" "Timer"(i16 0 ("Timer")) -> ()
                n239 = global write "Global 1.vi" "TCNT"(i16 0 ("Timer")) -> ()
              }
            }
          }
          frame -1 {
            n240 = global write "Global 1.vi" "Step"(w399) -> ()
          }
          frame 0, Default {
            w400 = 0.0 ("Vy")
            n241 = global write "Outputs.vi" "Vx"(w400) -> ()
            n242 = global write "Outputs.vi" "Vy"(w400) -> ()
            n243 = global write "Outputs.vi" "Vp"(w400) -> ()
          }
          frame 1 {
            n244 = call "Movement (SubVI).vi"("Speed"=w404, "Reset"=FALSE, "Acc"=10.0, "Goal P"=w405, "Goal Y"=w406, "Goal X"=w407) -> ("Vp"=w409:dbl, "Vy"=w410:dbl, "Vx"=w411:dbl, "Reach?"=w412:bool)  [unwired: 1 in]
            n245 = global write "Outputs.vi" "Vx"(w411) -> ()
            n246 = global write "Outputs.vi" "Vy"(w410) -> ()
            n247 = global write "Outputs.vi" "Vp"(w409) -> ()
            n248 = global read "Global 1.vi" "Step"() -> (w401:i16)
            n249 = Boolean To (0,1)(Boolean=w412) -> (0, 1=w413:i16)
            n250 = Add(x=w401, y=w413) -> (x+y=w402:i16)
            n251 = global write "Global 1.vi" "Step"(w402) -> ()
          }
          frame 2 {
            n252 = call "Set (SubVI).vi"("Mode"=w422, "speed"=40.0) -> ("Reach?"=w414:bool, "Vp"=w418:dbl, "Vy"=w419:dbl, "Vx"=w420:dbl)  [unwired: 4 in]
            n253 = global read "Global 1.vi" "Step"() -> (w415:i16)
            n254 = Boolean To (0,1)(Boolean=w414) -> (0, 1=w417:i16)
            n255 = global write "Outputs.vi" "Vx"(w420) -> ()
            n256 = global write "Outputs.vi" "Vy"(w419) -> ()
            n257 = global write "Outputs.vi" "Vp"(w418) -> ()
            n258 = Add(x=w415, y=w417) -> (x+y=w416:i16)
            n259 = global write "Global 1.vi" "Step"(w416) -> ()
          }
          frame 3 {
            n260 = global read "Global 1.vi" "Timer"() -> (w430:i16)
            n261 = case shown="0, Default" w430 {
              tunnel: w429 -> [_ w442 _]
              tunnel: w428 -> [_ w444 _]
              tunnel: w427 -> [_ w446 _]
              tunnel: w426 -> [_ w445 _]
              tunnel: w425 -> [_ w443 _]
              tunnel: w424 -> [_ w438 _]
              tunnel: w423 -> [_ w433 _]
              frame 0, Default {
                n262 = call "Tick Count"() -> ("Tick Count(mSec)"=w432:u32)
                n263 = global write "Global 1.vi" "Timer"(i16 1 ("Timer")) -> ()
                n264 = global write "Global 1.vi" "TCNT"(w432) -> ()
              }
              frame 1 {
                n265 = global read "Global 1.vi" "TCNT"() -> (w439:u64)
                n266 = call "Tick Count2"() -> ("Tick Count(mSec)"=w441:u32)
                n267 = call "arm_kinematics (SubVI).vi"("alpha"=w444, "y"=w446, "x"=w445) -> ("R"=w449:dbl, "alpha"=w448:dbl, "teta"=w447:dbl)
                n268 = Subtract(x=w441, y=w439) -> (x-y=w440:u64)
                n269 = global write "Outputs.vi" "Grip"(w443) -> ()
                n270 = global write "Outputs.vi" "alpha"(w448) -> ()
                n271 = global write "Outputs.vi" "J"(w433) -> ()
                n272 = global write "Outputs.vi" "teta"(w447) -> ()
                n273 = global write "Outputs.vi" "R"(w449) -> ()
                n274 = global write "Outputs.vi" "Z"(w442) -> ()
                n275 = Greater?(x=w440, y=w438) -> (0:w434:bool)
                n276 = global read "Global 1.vi" "Timer"() -> (w435:i16)
                n277 = Boolean To (0,1)(Boolean=w434) -> (0, 1=w437:i16)
                n278 = Add(x=w435, y=w437) -> (x+y=w436:i16)
                n279 = global write "Global 1.vi" "Timer"(w436) -> ()
              }
              frame 2 {
                n280 = global read "Global 1.vi" "Step"() -> (w452:i16)
                n281 = Increment(x=w452) -> (x+1=w453:i16)
                n282 = global write "Global 1.vi" "Step"(w453) -> ()
                n283 = global write "Global 1.vi" "Timer"(i16 0 ("Timer")) -> ()
                n284 = global write "Global 1.vi" "TCNT"(i16 0 ("Timer")) -> ()
              }
            }
          }
          frame 4 {
            n285 = global read "Global 1.vi" "V-x"() -> (w458:sgl)
            n286 = global read "Global 1.vi" "V-Ang"() -> (w456:sgl)
            n287 = global read "Global 1.vi" "V-y"() -> (w457:sgl)
            n288 = global read "Global 1.vi" "Timer"() -> (w459:i16)
            n289 = case shown="1" w459 {
              tunnel: w460 -> [_ w469 _]
              tunnel: w458 -> [_ w463 _]
              tunnel: w457 -> [_ w468 _]
              tunnel: w456 -> [_ w467 _]
              tunnel: w455 -> [_ w466 _]
              tunnel: w454 -> [_ w465 _]
              frame 0, Default {
                n290 = call "Tick Count3"() -> ("Tick Count(mSec)"=w462:u32)
                n291 = global write "Global 1.vi" "Timer"(i16 1 ("Timer")) -> ()
                n292 = global write "Global 1.vi" "TCNT"(w462) -> ()
              }
              frame 1 {
                n293 = global read "Global 1.vi" "TCNT"() -> (w474:u64)
                n294 = Not Equal To 0?(x=w463) -> (x != 0?=w464:bool)
                n295 = call "Tick Count4"() -> ("Tick Count(mSec)"=w476:u32)
                n296 = Subtract(x=w476, y=w474) -> (x-y=w475:u64)
                n297 = case shown="True" w464 {
                  tunnel: w463 -> [_ w481]
                  tunnel: w468 -> [_ w480]
                  tunnel: w467 -> [_ w479]
                  tunnel: w466 -> [_ w478]
                  tunnel: w465 -> [_ w477]
                  frame False {
                  }
                  frame True {
                    n298 = call "Rectangle Set (SubVI).vi"("x"=w481, "x in"=w478, "y"=w480, "alpha"=w479, "y in"=w477) -> ()  [unwired: 6 in]
                  }
                }
                n299 = Greater?(x=w475, y=w469) -> (0:w470:bool)
                n300 = global read "Global 1.vi" "Timer"() -> (w471:i16)
                n301 = Boolean To (0,1)(Boolean=w470) -> (0, 1=w473:i16)
                n302 = Add(x=w471, y=w473) -> (x+y=w472:i16)
                n303 = global write "Global 1.vi" "Timer"(w472) -> ()
              }
              frame 2 {
                n304 = global read "Global 1.vi" "Step"() -> (w484:i16)
                n305 = Increment(x=w484) -> (x+1=w485:i16)
                n306 = global write "Global 1.vi" "Step"(w485) -> ()
                n307 = global write "Global 1.vi" "Timer"(i16 0 ("Timer")) -> ()
                n308 = global write "Global 1.vi" "TCNT"(i16 0 ("Timer")) -> ()
              }
            }
          }
          frame 5 {
            n309 = global read "Global 1.vi" "Timer"() -> (w489:i16)
            n310 = case shown="1" w489 {
              tunnel: w488 -> [_ w494 _]
              tunnel: w487 -> [_ w493 _]
              tunnel: w486 -> [_ w492 _]
              frame 0, Default {
                n311 = call "Tick Count5"() -> ("Tick Count(mSec)"=w491:u32)
                n312 = global write "Global 1.vi" "Timer"(i16 1 ("Timer")) -> ()
                n313 = global write "Global 1.vi" "TCNT"(w491) -> ()
              }
              frame 1 {
                n314 = global read "Global 1.vi" "TCNT"() -> (w499:u64)
                n315 = call "Tick Count6"() -> ("Tick Count(mSec)"=w501:u32)
                n316 = global write "Outputs.vi" "Z"(w493) -> ()
                n317 = global write "Outputs.vi" "Grip"(w492) -> ()
                n318 = Subtract(x=w501, y=w499) -> (x-y=w500:u64)
                n319 = Greater?(x=w500, y=w494) -> (0:w495:bool)
                n320 = global read "Global 1.vi" "Timer"() -> (w496:i16)
                n321 = Boolean To (0,1)(Boolean=w495) -> (0, 1=w498:i16)
                n322 = Add(x=w496, y=w498) -> (x+y=w497:i16)
                n323 = global write "Global 1.vi" "Timer"(w497) -> ()
              }
              frame 2 {
                n324 = global read "Global 1.vi" "Step"() -> (w504:i16)
                n325 = Increment(x=w504) -> (x+1=w505:i16)
                n326 = global write "Global 1.vi" "Step"(w505) -> ()
                n327 = global write "Global 1.vi" "Timer"(i16 0 ("Timer")) -> ()
                n328 = global write "Global 1.vi" "TCNT"(i16 0 ("Timer")) -> ()
              }
            }
          }
          frame 6 {
            n329 = global read "Global 1.vi" "Timer"() -> (w508:i16)
            n330 = case shown="1" w508 {
              tunnel: w507 -> [_ w512 _]
              tunnel: w506 -> [_ w511 _]
              frame 0, Default {
                n331 = call "Tick Count11"() -> ("Tick Count(mSec)"=w510:u32)
                n332 = global write "Global 1.vi" "Timer"(i16 1 ("Timer")) -> ()
                n333 = global write "Global 1.vi" "TCNT"(w510) -> ()
              }
              frame 1 {
                n334 = global read "Global 1.vi" "TCNT"() -> (w517:u64)
                n335 = call "Tick Count12"() -> ("Tick Count(mSec)"=w519:u32)
                n336 = global write "Outputs.vi" "teta"(w511) -> ()
                n337 = Subtract(x=w519, y=w517) -> (x-y=w518:u64)
                n338 = Greater?(x=w518, y=w512) -> (0:w513:bool)
                n339 = global read "Global 1.vi" "Timer"() -> (w514:i16)
                n340 = Boolean To (0,1)(Boolean=w513) -> (0, 1=w516:i16)
                n341 = Add(x=w514, y=w516) -> (x+y=w515:i16)
                n342 = global write "Global 1.vi" "Timer"(w515) -> ()
              }
              frame 2 {
                n343 = global read "Global 1.vi" "Step"() -> (w522:i16)
                n344 = Increment(x=w522) -> (x+1=w523:i16)
                n345 = global write "Global 1.vi" "Step"(w523) -> ()
                n346 = global write "Global 1.vi" "Timer"(i16 0 ("Timer")) -> ()
                n347 = global write "Global 1.vi" "TCNT"(i16 0 ("Timer")) -> ()
              }
            }
          }
          frame 10 {
            n348 = global read "Global 1.vi" "Timer"() -> (w524:i16)
            n349 = case shown="1" w524 {
              tunnel: w525 -> [_ w528 _]
              frame 0, Default {
                n350 = call "Tick Count7"() -> ("Tick Count(mSec)"=w527:u32)
                n351 = global write "Global 1.vi" "Timer"(i16 1 ("Timer")) -> ()
                n352 = global write "Global 1.vi" "TCNT"(w527) -> ()
              }
              frame 1 {
                n353 = global read "Global 1.vi" "TCNT"() -> (w533:u64)
                n354 = call "Tick Count8"() -> ("Tick Count(mSec)"=w535:u32)
                n355 = Subtract(x=w535, y=w533) -> (x-y=w534:u64)
                n356 = Greater?(x=w534, y=w528) -> (0:w529:bool)
                n357 = global read "Global 1.vi" "Timer"() -> (w530:i16)
                n358 = Boolean To (0,1)(Boolean=w529) -> (0, 1=w532:i16)
                n359 = Add(x=w530, y=w532) -> (x+y=w531:i16)
                n360 = global write "Global 1.vi" "Timer"(w531) -> ()
              }
              frame 2 {
                n361 = global read "Global 1.vi" "Step"() -> (w538:i16)
                n362 = Increment(x=w538) -> (x+1=w539:i16)
                n363 = global write "Global 1.vi" "Step"(w539) -> ()
                n364 = global write "Global 1.vi" "Timer"(i16 0 ("Timer")) -> ()
                n365 = global write "Global 1.vi" "TCNT"(i16 0 ("Timer")) -> ()
              }
            }
          }
        }
        n366 = global read "Outputs.vi" "Vx"() -> (w360:dbl)
        n367 = global read "Outputs.vi" "Vy"() -> (w362:dbl)
        n368 = global read "Outputs.vi" "Vp"() -> (w361:dbl)
        n369 = global read "Inputs.vi" "C1/Encoder"() -> (w353:i32)
        n370 = global read "Inputs.vi" "C0/Encoder"() -> (w352:i32)
        n371 = global read "Inputs.vi" "B/Encoder"() -> (w351:i32)
        n372 = global read "Inputs.vi" "A/Encoder"() -> (w350:i32)
        n373 = call "Omni (SubVI).vi"("Vp"=w361, "Vy"=w362, "Vx"=w360) -> ("Back_Right"=w358:dbl, "Back_Left"=w363:dbl, "Front_Right"=w359:dbl, "Front_Left"=w356:dbl)  [unwired: 4 in]
        n374 = call "Front Left (SubVI).vi"("setpoint"=w356, "Counter Value"=w350, "error in"=w343) -> ("error out"=w357:errorcluster)  [unwired: 6 in, 1 out]
        n375 = call "Front Right (SubVI).vi"("error in"=w357, "Counter Value"=w351, "setpoint"=w359) -> ("error out"=w355:errorcluster)  [unwired: 7 in, 1 out]
        n376 = call "Back Left (SubVI).vi"("error in"=w355, "Counter Value"=w352, "setpoint"=w363) -> ("error out"=w354:errorcluster)  [unwired: 7 in, 1 out]
        n377 = call "Back Right (SubVI).vi"("error in"=w354, "Counter Value"=w353, "setpoint"=w358) -> ("error out"=w342:errorcluster)  [unwired: 7 in, 1 out]
        n378 = global read "Outputs.vi" "alpha"() -> (w344:i16)
        n379 = global read "Outputs.vi" "J"() -> (w345:i16)
        n380 = global read "Outputs.vi" "teta"() -> (w349:i16)
        n381 = global read "Outputs.vi" "R"() -> (w348:i16)
        n382 = global read "Outputs.vi" "Z"() -> (w347:i16)
        n383 = global read "Outputs.vi" "Grip"() -> (w346:i16)
        n384 = global read "Global 1.vi" "Stop"() -> (w373:bool)
        n385 = call "ARM Controller (SubVI).vi"("alpha"=w344, "Grip"=w346, "J"=w345, "error in (no error)"=w342, "Z"=w347, "R"=w348, "teta"=w349) -> ("error out"=w341:errorcluster)  [unwired: 4 in]
        n386 = Or(x=w341, y=w373) -> (x .or. y?=w381:bool)
      }
      n387 = while {
        stop <- "Stop" stop-if-true
        n388 = global write "Global 1.vi" "Stop"("Stop") -> ()
      }
      n389 = node-c288(w118) -> ()
      n390 = Merge Errors(w112, w113) -> (w114:errorcluster)
    }
    frame #3 {
      # "Close"
      n391 = call <vilib>:"Reset myRIO.vi"("error in (no error)"=w545) -> ("error out"=→"error out":errorcluster)  [unwired: 10 in]
    }
  }
